vi "subvi_PointerToDataAsByteArray.vi"(8 "error in (no error)":errorcluster, 10 "Size":i32, 11 "Pointer":i32) -> (0 "error out":errorcluster, 3 "Byte Array Out":u8[](array[numeric]))   [LabVIEW 2013]
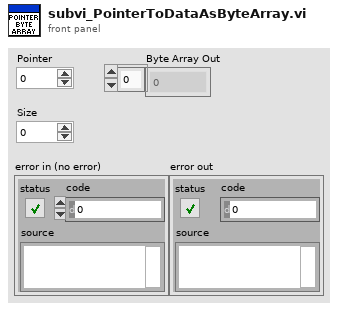
[diagram p1: front panel]
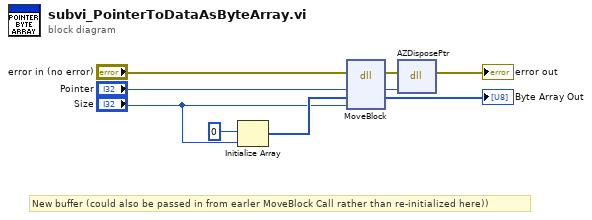
[diagram p0: block diagram]
diagram:
  # "New buffer (could also be passed in from earler MoveBlock Call rather than re-initialized here))"
  n1 = Initialize Array(u8 0, "Size") -> (w9:u8[])
  n2 = dll-call lib="LabVIEW" fn="MoveBlock"(error in="error in (no error)", "src"="Pointer", "dest"=w9, "size"="Size") -> (error out=w4:errorcluster, "src"=w3:i32, "dest"=→"Byte Array Out":u8[])  [unwired: 4 in, 1 out]
  n3 = dll-call lib="LabVIEW" fn="AZDisposePtr"(error in=w4, "ptr"=w3) -> (error out=→"error out":errorcluster)  [unwired: 4 in, 1 out]
